vi "evo irimager tcp init.vi"(8 "port":i32, 10 "ip":string) -> (0 "h out":i32, 1 "w out":i32, 3 "function return 2":i32)   [LabVIEW 2025, in "libirimager_direct_binding.lvlib"]
doc: "DIRECT_API int evo_irimager_tcp_init(const char* ip, int port);"
uses:
  libirimager_direct_binding.lvlib
  labview/libirimager.dll
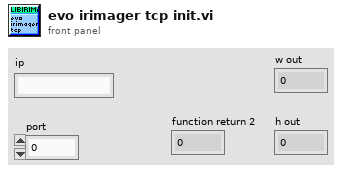
[diagram p1: front panel]
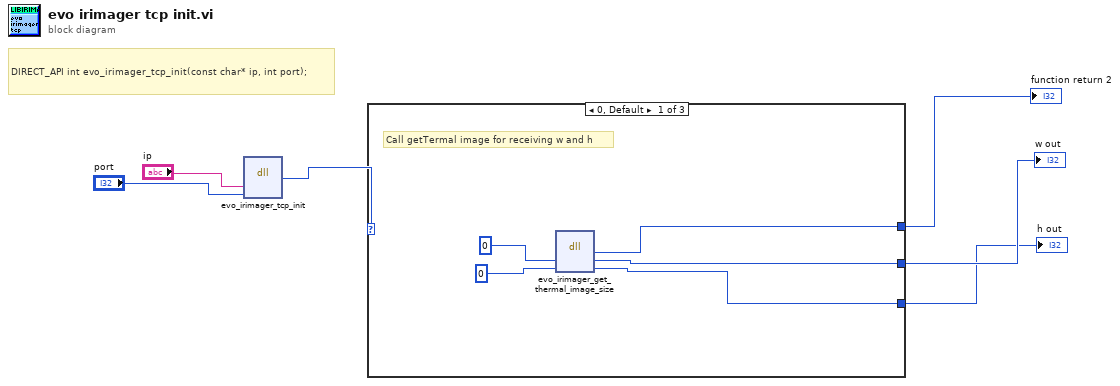
[diagram p0: block diagram]
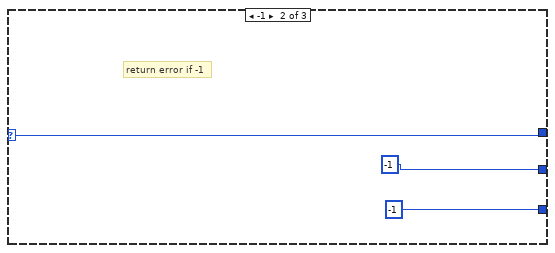
[diagram p2: hidden frame]
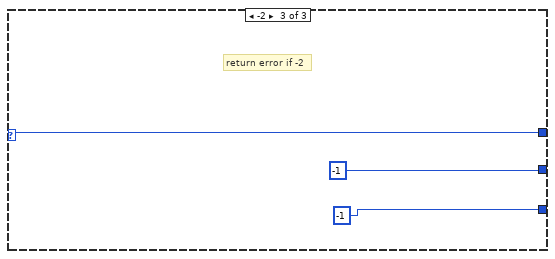
[diagram p3: hidden frame]
diagram:
  # "DIRECT_API int evo_irimager_tcp_init(const char* ip, int port);"
  n1 = dll-call lib="C:/Users/HelmutEngelhardt/Documents/labview/libirimager.dll" fn="evo_irimager_tcp_init"("ip"="ip", "port"="port") -> ("Rückgabetyp"=w1:i32)  [unwired: 5 in, 2 out]
  n2 = case shown="0, Default" w1 {
    selector: w1 -> [_ w14 w17]
    tunnel: [w10 -1 -1] -> w6
    tunnel: [w9 -1 -1] -> w5
    tunnel: [w11 w14 w17] -> w4
    frame 0, Default {
      # "Call getTermal image for receiving w and h"
      n3 = dll-call lib="C:/Users/HelmutEngelhardt/Documents/labview/libirimager.dll" fn="evo_irimager_get_thermal_image_size"("w"=0, "h"=0) -> ("Rückgabetyp"=w11:i32, "w"=w10:i32, "h"=w9:i32)  [unwired: 3 in, 2 out]
    }
    frame -1 {
      # "return error if -1"
    }
    frame -2 {
      # "return error if -2"
    }
  }
  "function return 2" <- w4
  "w out" <- w6
  "h out" <- w5
